vi "Read Notifier Ref.vi"(8 "error in":errorcluster, 11 "NotifierMessageTransport in":refnum<class "NotifierMessageTransport.lvclass">) -> (0 "error out":errorcluster, 2 "Notifier Ref":refnum<notifier>, 3 "NotifierMessageTransport out":refnum<class "NotifierMessageTransport.lvclass">)   [LabVIEW 2016, in "NotifierMessageTransport.lvclass"]
uses:
  NotifierMessageTransport.lvclass
  IMessagePayload/IMessagePayload.lvclass
  NotifierMessageTransport.lvclass/NotifierMessageTransport.ctl
panel:
  # "INPUTS"
  # "OUTPUTS"
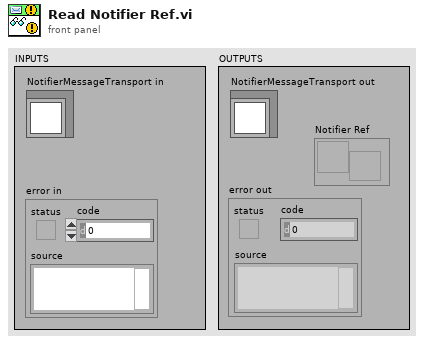
[diagram p1: front panel]
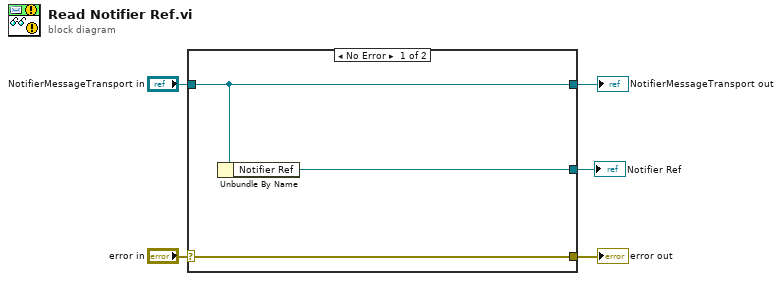
[diagram p0: block diagram]
diagram:
  n1 = case shown="No Error" "error in" {
    selector: "error in" -> [w8 w9]
    tunnel: [w8 w9] -> w4
    tunnel: [w7 w10] -> w2
    tunnel: "NotifierMessageTransport in" -> [w7 w10]
    tunnel: [w6 _] -> w1
    frame No Error {
      n2 = Unbundle By Name(w7) -> ("Notifier Ref"=w6:refnum<notifier>)
    }
    frame Error {
    }
  }
  "error out" <- w4
  "NotifierMessageTransport out" <- w2
  "Notifier Ref" <- w1
